vi "Init.vi"(8 "error in":errorcluster, 11 "Data in":T1) -> (0 "error out":errorcluster, 3 "Data out":T1)   [LabVIEW 2020, in "AR Example.lvlib"]
uses:
  AR Example.lvlib
  Data.ctl
  g_ar_toolkit.capture/CameraManager/CameraManager.lvclass
  Tab Control.ctl
  State.ctl
  Global Events.ctl
  <vilib>/Utility/miscctls.llb/LVPointTypeDef.ctl
  8e44b1d0-1089-4c98-a43f-40977132d2da.vi
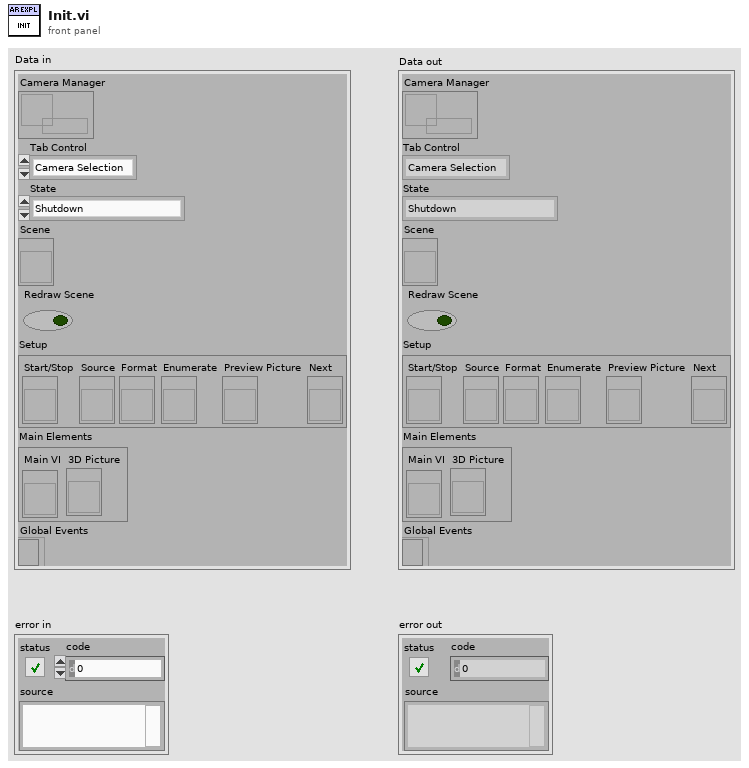
[diagram p1: front panel]
types:
  T1 = typedef "AR Example.lvlib/Data.ctl" = cluster{"Camera Manager":refnum<data-value>, "Tab Control":T2, "State":T3, "Scene":refnum<vi>, "Redraw Scene":bool, "Setup":cluster{"Start/Stop":refnum<vi>, "Source":refnum<vi>, "Format":refnum<vi>, "Enumerate":refnum<vi>, "Preview Picture":refnum<vi>, "Next":refnum<vi>}, "Main Elements":cluster{"Main VI":refnum<vi>, "3D Picture":refnum<vi>}, "Global Events":T4}
  T2 = typedef "AR Example.lvlib/Tab Control.ctl" = enum8{"Camera Selection"}
  T3 = typedef "AR Example.lvlib/State.ctl" = enum16{"Shutdown", "Initialize", "Select Camera"}
  T4 = typedef "AR Example.lvlib/Global Events.ctl" = refnum<event-registration>
  T5 = enum16{"Global Events", "Default Values", "Pane Origins", "Camera Manager", "Enumerate Cameras", "State"}
  T6 = enum16{"Global Events", "Default Values", "Pane Origins", "Camera Manager", "Enumerate Cameras", "State"}[]
  T7 = typedef "LVPointTypeDef.ctl" = cluster{"Horizontal":i16, "Vertical":i16}
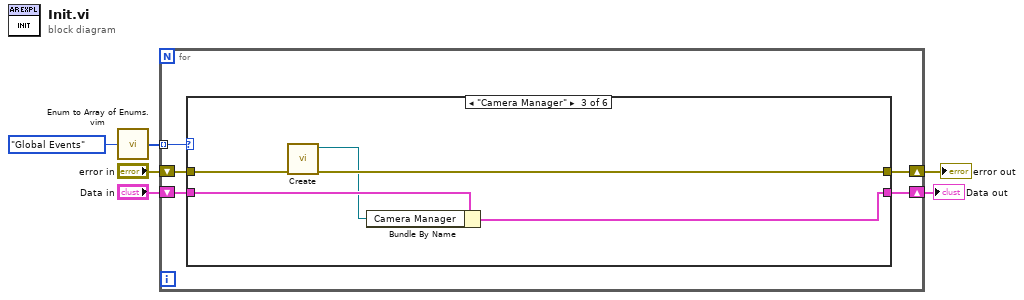
[diagram p0: block diagram]
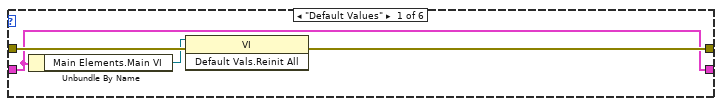
[diagram p2: hidden frame]
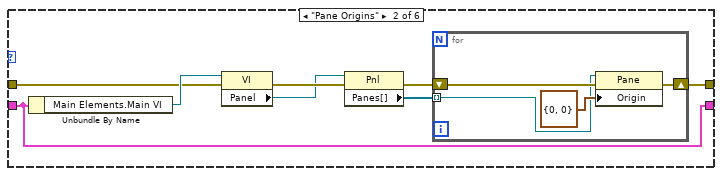
[diagram p3: hidden frame]
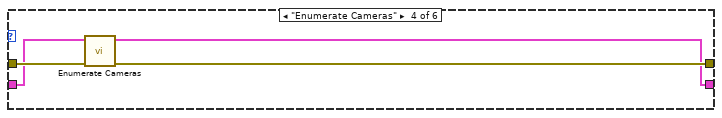
[diagram p4: hidden frame]
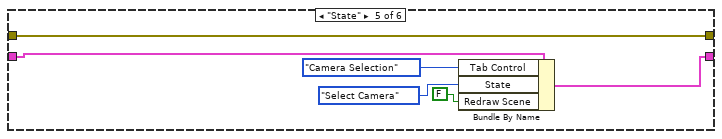
[diagram p5: hidden frame]
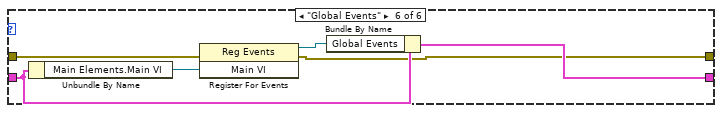
[diagram p6: hidden frame]
diagram:
  n1 = call "Enum to Array of Enums.vim"("enum"=T5."Global Events") -> ("array of enums"=w4:T6)
  n2 = for {
    tunnel: w4 -> [w11] mode=indexing
    shift-right: [w7] -> w1
    shift-left: "Data in" -> [w10]
    shift-right: [w8] -> w2
    shift-left: "error in" -> [w9]
    n3 = case shown="\"Camera Manager\"" w11 {
      tunnel: [w15 w16 w29 w34 w37 w44] -> w8
      tunnel: w10 -> [w13 w23 w31 w35 w42 w47]
      tunnel: w9 -> [w14 w19 w32 w36 w37 w43]
      tunnel: [w13 w23 w30 w33 w38 w48] -> w7
      frame "Default Values" {
        n4 = Unbundle By Name(w13) -> ("Main Elements.Main VI"=w12:refnum<vi>)
        n5 = invoke class="VI" method="Default Vals.Reinit All"(reference=w12, error in=w14) -> (error out=w15:errorcluster)  [unwired: 1 in, 2 out]
      }
      frame "Pane Origins" {
        n6 = Unbundle By Name(w23) -> ("Main Elements.Main VI"=w20:refnum<vi>)
        n7 = property class="VI"(reference=w20, error in=w19) -> (error out=w22:errorcluster, "Panel"=w21:refnum<vi>)  [unwired: 1 out]
        n8 = property class="Pnl"(reference=w21, error in=w22) -> (error out=w18:errorcluster, "Panes[]"=w17:refnum<vi>[])  [unwired: 1 out]
        n9 = for {
          shift-right: [w24] -> w16
          shift-left: w18 -> [w26]
          tunnel: w17 -> [w25] mode=indexing
          n10 = property class="Pane"(reference=w25, error in=w26, "Origin"=T7 {"Horizontal"=0, "Vertical"=0}) -> (error out=w24:errorcluster)  [unwired: 1 out]
        }
      }
      frame "Camera Manager" {
        n11 = call "Create.vi"("error in (no error)"=w32) -> ("error out"=w29:errorcluster, "CameraManager"=w28:refnum<data-value>)  [unwired: 9 in]
        n12 = Bundle By Name(cluster=w31, "Camera Manager"=w28) -> (w30:T1)
      }
      frame "Enumerate Cameras" {
        n13 = call "Enumerate Cameras.vi"("error in"=w36, "Data in"=w35) -> ("error out"=w34:errorcluster, "Data out"=w33:T1)  [unwired: 8 in]
      }
      frame "State" {
        n14 = Bundle By Name(cluster=w42, "Tab Control"=Tab_Control."Camera Selection", "State"=State."Select Camera", "Redraw Scene"=FALSE) -> (w38:T1)
      }
      frame "Global Events" {
        n15 = Unbundle By Name(w47) -> ("Main Elements.Main VI"=w46:refnum<vi>)
        n16 = register-events(error in=w43, w46) -> (reference out=w45:refnum<event-registration>, error out=w44:errorcluster)  [unwired: 1 in]
        n17 = Bundle By Name(cluster=w47, "Global Events"=w45) -> (w48:T1)
      }
    }
  }
  "error out" <- w2
  "Data out" <- w1
